vi "Validate Table Name.vi"(8 "error in":errorcluster, 11 "Table Name in":string) -> (0 "error out":errorcluster, 3 "Table Name out":string)   [LabVIEW 2019, in "Open Xml.lvlib"]
uses:
  Open Xml.lvlib
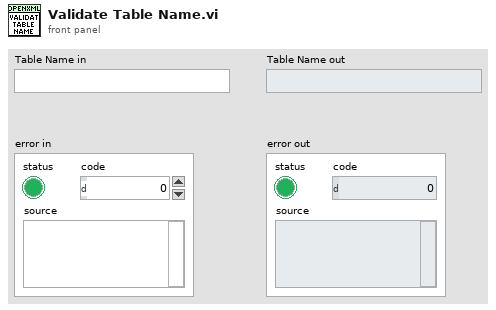
[diagram p1: front panel]
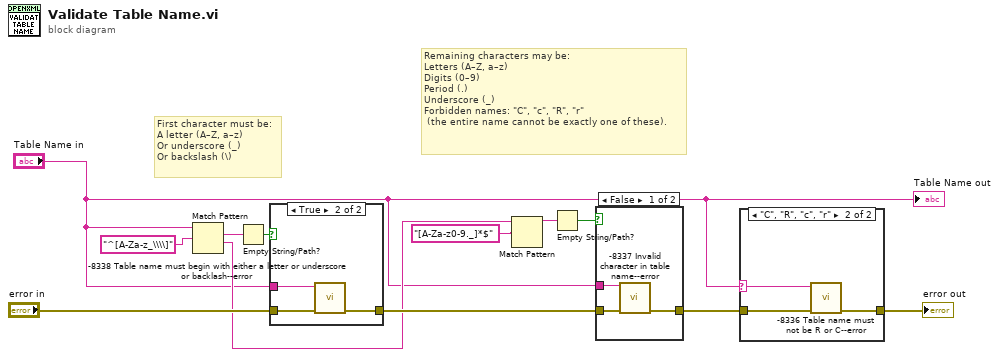
[diagram p0: block diagram]
diagram:
  # "Remaining characters may be:\nLetters (A–Z, a–z)\nDigits (0–9)\nPeriod (.)\nUnderscore (_)\nForbidden names: \"C\", \"c\", \"R\", \"r\"\n (the entire name cannot be exactly one of these)."
  # "First character must be:\nA letter (A–Z, a–z)\nOr underscore (_)\nOr backslash (\\)"
  n1 = Match Pattern(string="Table Name in", regular expression="^[A-Za-z_\\\\]") -> (match substring=w9:string, after substring=w7:string)  [unwired: 1 in, 2 out]
  n2 = Empty String/Path?(string/path=w9) -> (empty?=w8:bool)
  n3 = case shown="True" w8 {
    tunnel: "error in" -> [w13 w16]
    tunnel: [w13 w15] -> w11
    tunnel: "Table Name in" -> [_ w14]
    frame False {
    }
    frame True {
      n4 = call "-8338 Table name must begin with either a letter or underscore or backlash--error.vi"("error in"=w16, "Argument"=w14) -> ("error out"=w15:errorcluster)  [unwired: 8 in, 1 out]
    }
  }
  n5 = Match Pattern(string=w7, regular expression="[A-Za-z0-9._]*$") -> (before substring=w2:string)  [unwired: 1 in, 3 out]
  n6 = Empty String/Path?(string/path=w2) -> (empty?=w6:bool)
  n7 = case shown="False" w6 {
    tunnel: w11 -> [w19 w20]
    tunnel: [w18 w20] -> w4
    tunnel: "Table Name in" -> [w17 _]
    frame False {
      n8 = call "-8337 Invalid character in table name--error.vi"("error in"=w19, "Argument"=w17) -> ("error out"=w18:errorcluster)  [unwired: 8 in, 1 out]
    }
    frame True {
    }
  }
  n9 = case shown="\"C\", \"R\", \"c\", \"r\"" "Table Name in" {
    selector: "Table Name in" -> [_ w22]
    tunnel: w4 -> [w21 w24]
    tunnel: [w21 w23] -> w3
    frame "False", Default {
    }
    frame "C", "R", "c", "r" {
      n10 = call "-8336 Table name must not be R or C--error.vi"("error in"=w24, "Argument"=w22) -> ("error out"=w23:errorcluster)  [unwired: 8 in, 1 out]
    }
  }
  "error out" <- w3
  "Table Name out" <- "Table Name in"
